vi "Send DC.vi"() -> ()   [LabVIEW 2020]
uses:
  Binary Array Server DAQmx 4 Apr 2016.llb/DataSocketCluster.ctl
  2532044f-97d0-4a93-887a-290feb254d97.vi
  <vilib>/Comparison/Less/Less Functor/Less Functor.lvclass
panel:
  out "sorted array":dbl[](array[numeric])
  out "Segmenst in array":dbl[](array[numeric]) format="%#_16g"
  out "Segment String":string
  in  "TimeOut Time (s)":dbl=5.0 format="%.2f"
  in  "Count in":i32
  out "error out":errorcluster
  in  "error in (no error)":errorcluster
  in  "DataSocketCluster In":T1={"Server Machine"="siskin", "Client Machine"="becard", "Data"="P2", "TimeStamp"=0.0, "Count"=0, "Target Process"="General Server"} {"TimeStamp" format="%.2f"}
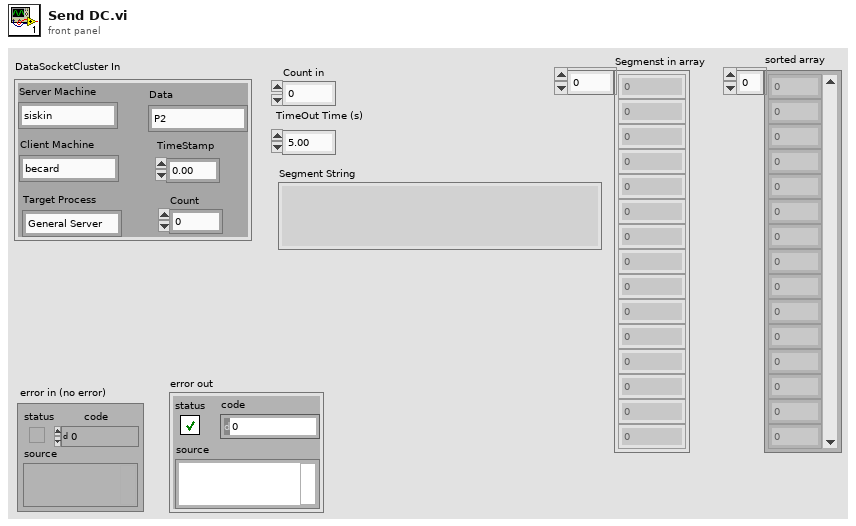
[diagram p1: front panel]
types:
  T1 = typedef "DataSocketCluster.ctl" = cluster{"Server Machine":string, "Client Machine":string, "Data":string, "TimeStamp":dbl, "Count":i32, "Target Process":string}
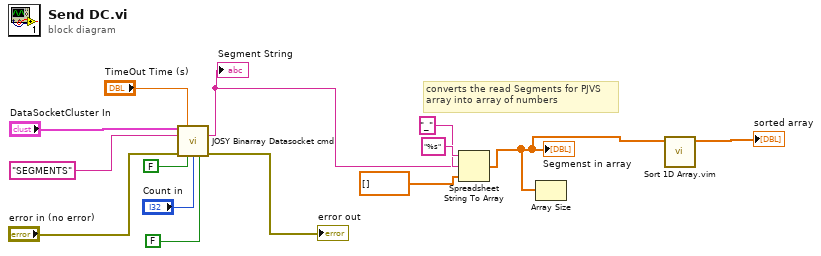
[diagram p0: block diagram]
diagram:
  # "converts the read Segments for PJVS\narray into array of numbers"
  n1 = call "JOSY Binarray Datasocket cmd.vi"("DataSocketCluster In"="DataSocketCluster In", "TimeOut Time (s)"="TimeOut Time (s)", "Command"="SEGMENTS", "error in (no error)"="error in (no error)", "Command has variable"=FALSE, "Count in"="Count in", "String"=FALSE) -> ("Reply data"=w3:string, "error out"=→"error out":errorcluster)  [unwired: 5 in, 2 out]
  "Segment String" <- w3
  n2 = Spreadsheet String To Array(delimiter (Tab)="_", format string="%s", spreadsheet string=w3, array type (2D Dbl)=dbl[] []) -> (array=w2:dbl[])
  "Segmenst in array" <- w2
  n3 = Array Size(array=w2) -> ()  [unwired: 1 out]
  n4 = call "Sort 1D Array.vim"("unsorted array"=w2) -> ("sorted array"=→"sorted array":dbl[])  [unwired: 10 in]
